vi "CRYInit One Data.vi"(8 "Waveform In":T1={"Waveform"={"X0"=0.0, "dX"=0.0, "Y"=[]}, "X data"=1, "Y data"=1, "Y axis"=1, "X unit"="s", "Y unit"="s", "Y dB ref"=1.0, "display Y"=TRUE, "display X"=TRUE, "Overload?"=TRUE, "Test Info"="", "Step No."=0, "Name"="", "protected"=FALSE, "Sqc history"=[], "Signal Channel ID"=0, "Plot Settings"={"Color"=0, "Interpolation"=0, "Point Style"=0, "Line Style"=0, "Point Color"=0, "Line Width"=0, "Bar Plot Style"=0, "Fill To"=0}, "AutoProtect"=FALSE} {"Y dB ref" format="%.1f"; "Y axis" items=["Log", "Lin"]; "Y data" items=["dB", "Lin"]; "X data" items=["dB", "Lin"]}, 9 "Result In":T2={"Name"="Test for Signal [L]", "Margin"=nan, "unit"="", "Verdict"=FALSE, "Limit"="", "Max/Min"="", "protected"=FALSE, "Step No."=0, "Test Info"="", "AutoProtect"=FALSE} {"Margin" format="%.2f"}, 10 "Data In":T3={"Name"="", "Curve"=[], "X data"=1, "Y data"=1, "Z data"=1, "X axis"=0, "Y axis"=1, "Z axis"=1, "X unit"="Hz", "Y unit"="", "Z unit"="deg.", "X dB ref"=1.0, "Y dB ref"=1.0, "Z dB ref"=1.0, "single val"=FALSE, "protected"=FALSE, "display X"=TRUE, "display Y"=TRUE, "display Z"=TRUE, "Test Info"="", "Step No."=0, "Plot Settings"={"Color"=0, "Interpolation"=0, "Point Style"=0, "Line Style"=0, "Point Color"=0, "Line Width"=0, "Bar Plot Style"=0, "Fill To"=0}, "AutoProtect"=FALSE} {"Z data" items=["dB", "Lin"]; "X data" items=["dB", "Lin"]; "Y data" items=["dB", "Lin"]; "Z dB ref" format="%.1f"; "Z axis" items=["Log", "Lin"]; "X dB ref" format="%.1f"; "X axis" items=["Log", "Lin"]; "Y axis" items=["Log", "Lin"]; "Y dB ref" format="%.1f"; "Curve"."z" format="%.2f"; "Curve"."y" format="%.2f"; "Curve"."x" format="%.2f"}, 11 "Type":enum16{"Curves", "Values", "Results", "WFM"}(ring)) -> (0 "Waveform Out":T1={"Waveform"={"X0"=0.0, "dX"=0.0, "Y"=[]}, "X data"=1, "Y data"=1, "Y axis"=1, "X unit"="s", "Y unit"="s", "Y dB ref"=1.0, "display Y"=TRUE, "display X"=TRUE, "Overload?"=TRUE, "Test Info"="", "Step No."=0, "Name"="", "protected"=FALSE, "Sqc history"=[], "Signal Channel ID"=0, "Plot Settings"={"Color"=0, "Interpolation"=0, "Point Style"=0, "Line Style"=0, "Point Color"=0, "Line Width"=0, "Bar Plot Style"=0, "Fill To"=0}, "AutoProtect"=FALSE} {"Y dB ref" format="%.1f"; "Y axis" items=["Log", "Lin"]; "Y data" items=["dB", "Lin"]; "X data" items=["dB", "Lin"]}, 1 "Result Out":T2={"Name"="Test for Signal [L]", "Margin"=nan, "unit"="", "Verdict"=FALSE, "Limit"="", "Max/Min"="", "protected"=FALSE, "Step No."=0, "Test Info"="", "AutoProtect"=FALSE} {"Margin" format="%.2f"}, 2 "Data Out":T3={"Name"="", "Curve"=[], "X data"=1, "Y data"=1, "Z data"=1, "X axis"=0, "Y axis"=1, "Z axis"=1, "X unit"="Hz", "Y unit"="", "Z unit"="deg.", "X dB ref"=1.0, "Y dB ref"=1.0, "Z dB ref"=1.0, "single val"=FALSE, "protected"=FALSE, "display X"=TRUE, "display Y"=TRUE, "display Z"=TRUE, "Test Info"="", "Step No."=0, "Plot Settings"={"Color"=0, "Interpolation"=0, "Point Style"=0, "Line Style"=0, "Point Color"=0, "Line Width"=0, "Bar Plot Style"=0, "Fill To"=0}, "AutoProtect"=FALSE} {"Z data" items=["dB", "Lin"]; "X data" items=["dB", "Lin"]; "Y data" items=["dB", "Lin"]; "Z dB ref" format="%.1f"; "Z axis" items=["Log", "Lin"]; "X dB ref" format="%.1f"; "X axis" items=["Log", "Lin"]; "Y axis" items=["Log", "Lin"]; "Y dB ref" format="%.1f"; "Curve"."z" format="%.2f"; "Curve"."y" format="%.2f"; "Curve"."x" format="%.2f"})   [LabVIEW 2013]
uses:
  CRYSystem/Typedef Control/CRYData Cluster.ctl
  CRYSystem/Typedef Control/CRYResult Cluster.ctl
  CRYSystem/Typedef Control/CRYWaveform Cluster.ctl
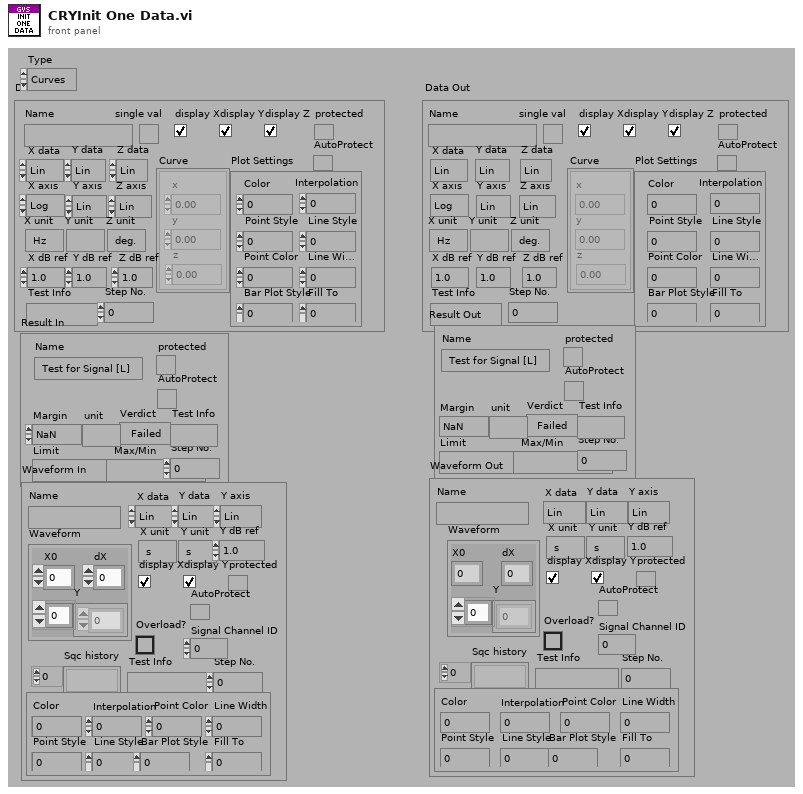
[diagram p1: front panel]
types:
  T1 = typedef "CRYWaveform Cluster.ctl" = cluster{"Waveform":cluster{"X0":dbl, "dX":dbl, "Y":sgl[]}, "X data":u16, "Y data":u16, "Y axis":u16, "X unit":string, "Y unit":string, "Y dB ref":dbl, "display Y":bool, "display X":bool, "Overload?":bool, "Test Info":string, "Step No.":i32, "Name":string, "protected":bool, "Sqc history":string[], "Signal Channel ID":i32, "Plot Settings":cluster{"Color":u32, "Interpolation":u8, "Point Style":u8, "Line Style":u8, "Point Color":u32, "Line Width":u8, "Bar Plot Style":u8, "Fill To":i16}, "AutoProtect":bool}
  T2 = typedef "CRYResult Cluster.ctl" = cluster{"Name":string, "Margin":dbl, "unit":string, "Verdict":bool, "Limit":string, "Max/Min":string, "protected":bool, "Step No.":i32, "Test Info":string, "AutoProtect":bool}
  T3 = typedef "CRYData Cluster.ctl" = cluster{"Name":string, "Curve":cluster{"x":dbl, "y":dbl, "z":dbl}[], "X data":u16, "Y data":u16, "Z data":u16, "X axis":u16, "Y axis":u16, "Z axis":u16, "X unit":string, "Y unit":string, "Z unit":string, "X dB ref":dbl, "Y dB ref":dbl, "Z dB ref":dbl, "single val":bool, "protected":bool, "display X":bool, "display Y":bool, "display Z":bool, "Test Info":string, "Step No.":i32, "Plot Settings":cluster{"Color":u32, "Interpolation":u8, "Point Style":u8, "Line Style":u8, "Point Color":u32, "Line Width":u8, "Bar Plot Style":u8, "Fill To":i16}, "AutoProtect":bool}
  T4 = cluster{"freq":dbl, "ampl":dbl, "cycles":dbl, "samples":i32}[]
  T5 = typedef "CRYStimulus Test Infor Cluster.ctl" = cluster{"Stimulus Type":string, "Signal Type":string, "In/Out":bool, "FAPS":cluster{"freq":dbl, "ampl":dbl, "cycles":dbl, "samples":i32}[], "Sampling Rate":dbl, "Samples":i32, "Analysis Param":string, "Resolution":u16, "Steps":u32, "Analysis Value":dbl[], "Diff Freq":dbl, "FStart":dbl, "FStop":dbl, "Calibration Param":string, "Anti Alias":dbl, "Level Out1":dbl, "Level Out2":dbl, "EQ":bool}
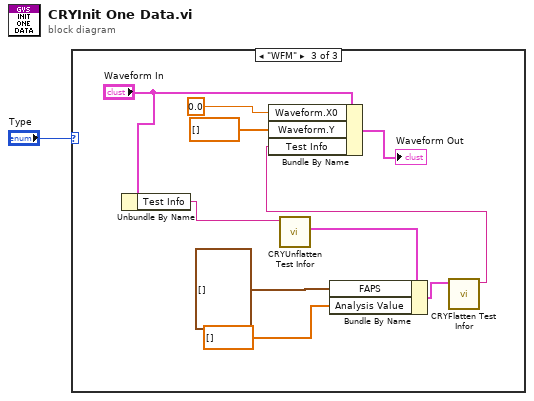
[diagram p0: block diagram]
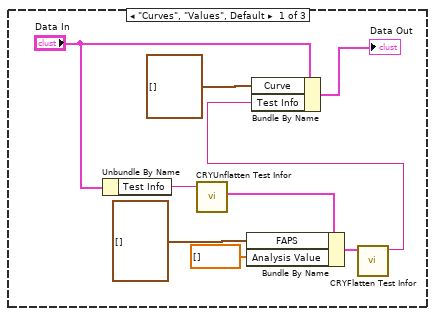
[diagram p2: hidden frame]
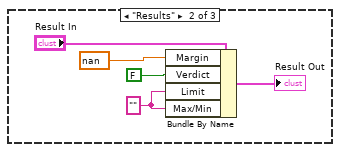
[diagram p3: hidden frame]
diagram:
  n1 = case shown="\"WFM\"" "Type" {
    frame "Curves", "Values", Default {
      n2 = Unbundle By Name("Data In") -> ("Test Info"=w8:string)
      n3 = call "CRYUnflatten Test Infor.vi"("Falattend test infor"=w8) -> ("unflattened test infor data"=w7:T5)  [unwired: 8 in, 1 out]
      n4 = Bundle By Name(cluster=w7, "FAPS"=T4 [], "Analysis Value"=dbl[] []) -> (w5:T5)
      n5 = call "CRYFlatten Test Infor.vi"("Test Infor data"=w5) -> ("Fattened Data"=w3:string)  [unwired: 10 in]
      n6 = Bundle By Name(cluster="Data In", "Curve"=cluster{"x":dbl, "y":dbl, "z":dbl}[] [], "Test Info"=w3) -> (→"Data Out":T3)
    }
    frame "Results" {
      w12 = "" ("Limit")
      n7 = Bundle By Name(cluster="Result In", "Margin"=nan, "Verdict"=FALSE, "Limit"=w12, "Max/Min"=w12) -> (→"Result Out":T2)
    }
    frame "WFM" {
      n8 = Unbundle By Name("Waveform In") -> ("Test Info"=w21:string)
      n9 = call "CRYUnflatten Test Infor.vi"("Falattend test infor"=w21) -> ("unflattened test infor data"=w20:T5)  [unwired: 8 in, 1 out]
      n10 = Bundle By Name(cluster=w20, "FAPS"=T4 [], "Analysis Value"=dbl[] []) -> (w17:T5)
      n11 = call "CRYFlatten Test Infor.vi"("Test Infor data"=w17) -> ("Fattened Data"=w16:string)  [unwired: 10 in]
      n12 = Bundle By Name(cluster="Waveform In", "Waveform.X0"=0.0 ("Waveform.dX"), "Waveform.Y"=sgl[] [], "Test Info"=w16) -> (→"Waveform Out":T1)
    }
  }
